vi "Uninitialize.vi"(8 "error in (no error)":errorcluster, 11 "Device in":refnum<class "Device.lvclass">) -> (0 "error out":errorcluster, 3 "Device out":refnum<class "Device.lvclass">)   [LabVIEW 2017, in "Device.lvclass"]
uses:
  Device.lvclass
  Typedefs/PublicEvents--Device.Uninitialized.ctl
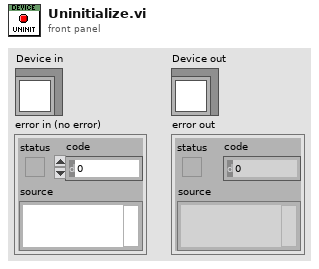
[diagram p1: front panel]
types:
  T1 = typedef "Device.lvclass/PublicEvents--Device.Uninitialized.ctl" = bool
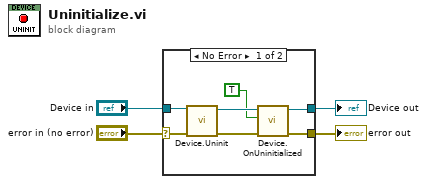
[diagram p0: block diagram]
diagram:
  n1 = case shown="No Error" "error in (no error)" {
    selector: "error in (no error)" -> [w10 w13]
    tunnel: [w6 w13] -> w3
    tunnel: [w7 w12] -> w1
    tunnel: "Device in" -> [w11 w12]
    frame No Error {
      n2 = call-dynamic "Device.Uninit.vi"("error in (no error)"=w10, "Device in"=w11) -> ("error out"=w8:errorcluster, "Device out"=w9:refnum<class "Device.lvclass">)  [unwired: 8 in]
      n3 = call "Device.OnUninitialized.vi"("error in (no error)"=w8, "Result"=T1 TRUE, "Device in"=w9) -> ("error out"=w6:errorcluster, "Device out"=w7:refnum<class "Device.lvclass">)  [unwired: 7 in]
    }
    frame Error {
    }
  }
  "error out" <- w3
  "Device out" <- w1
